vi "Get Minimum Import Pulse Width (clocks).vi"(0 "import signal":T1, 2 "acq":refnum<class "niUSRP DSP v2 FPGA.lvclass">=refnum) -> (4 "minimum import pulse width (clocks)":u16)   [LabVIEW 2023]
doc: "this setting determines how long the minimum pulse duration is for an exported signal. to calculate what the value is in seconds take the reciprocal of the ADC/DAC rate (seconds per clock tick) and multiply by number of clocks (min event pulse width)."
uses:
  <vilib>/rvi/DataTransferAndStorage/Container/XNode/niFpgaContainer.xnode
  <vilib>/rvi/DataTransferAndStorage/Register/Emulation/niFpgaRegisterEmulationRefIn.vi
  <instrlib>/niVST/Reference FPGA/FPGA/ACQ DSP/niUSRP DSP v2 FPGA.lvclass
  <instrlib>/niVST/Reference FPGA/FPGA/Acquisition/v1/Registers/Public/Typedefs/Imported Signals.ctl
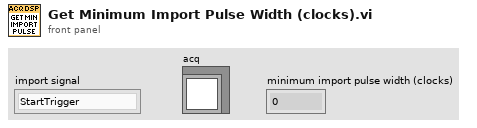
[diagram p1: front panel]
types:
  T1 = typedef "niVST Acquisition Registers v1 FPGA.lvclass/Imported Signals.ctl" = enum16{"StartTrigger", "RefTrigger", "AdvTrigger", "Configuration List Step Trigger", "Timer Start Trigger"}
  T2 = typedef "niUSRP DSP v2 FPGA.lvclass/DSP Shared Regs.ctl" = cluster{"rfsa.abort":refnum<k21>, "reset":refnum<k21>, "reset.done":refnum<k21>, "inject data into path":refnum<k21>, "data has entered path":refnum<k21>, "ADC overrange I":refnum<k21>, "ADC overrange Q":refnum<k21>, "ADC overrange.clear":refnum<k21>, "overflow":refnum<k21>, "overflow.clear":refnum<k21>, "pipeline delay":refnum<k21>, "group delay (output samples)":refnum<k21>, "dynamic delay.data clock ticks":refnum<k21>, "dynamic delay.samples":refnum<k21>, "scale data by 2":refnum<k21>, "bypass additional group delay":refnum<k21>, "debug.use wrapback data":refnum<k21>}
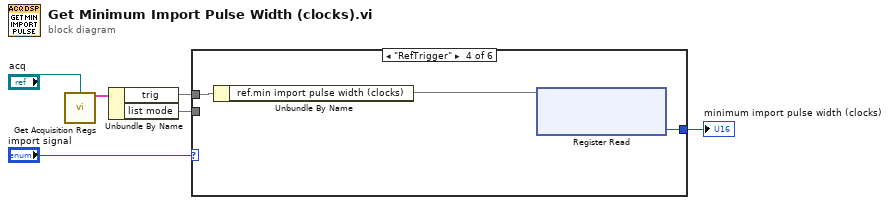
[diagram p0: block diagram]
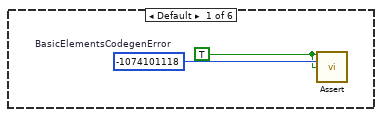
[diagram p2: hidden frame]
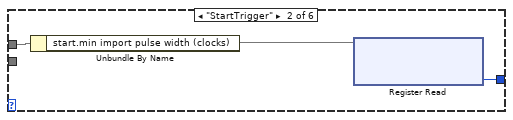
[diagram p3: hidden frame]
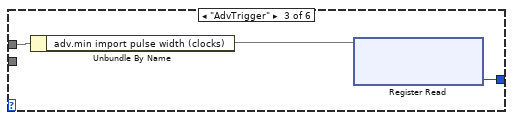
[diagram p4: hidden frame]
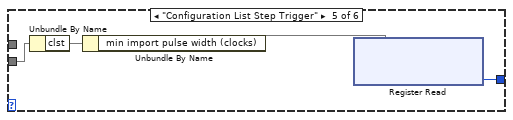
[diagram p5: hidden frame]
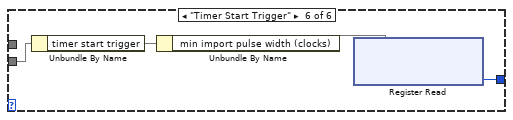
[diagram p6: hidden frame]
diagram:
  n1 = call-dynamic "Get Acquisition Regs.vi"("acq"="acq") -> ("dsp"=w3:T2)  [unwired: 14 in]
  n2 = Unbundle By Name(w3) -> ("trig"=w4, "list mode"=w1)
  n3 = case shown="\"RefTrigger\"" "import signal" {
    tunnel: [_ w10 w13 w16 w18 w22] -> w6
    tunnel: w4 -> [_ w9 w12 w15 _ _]
    tunnel: w1 -> [_ _ _ _ w21 w25]
    frame Default {
      w7 = TRUE ("assert")
      w8 = -1074101118  # BasicElementsCodegenError
      n4 = call <instrlib>:"Assert.vi"("assert"=w7, "error code"=w8, "enable show error"=w7) -> ()  [unwired: 13 in]
    }
    frame "StartTrigger" {
      n5 = Unbundle By Name(w9) -> ("start.min import pulse width (clocks)"=w11)
      n6 = xnode ("Register Read")("Register In"=w11) -> ("Data"=w10:u16)  [unwired: 1 out]
    }
    frame "AdvTrigger" {
      n7 = Unbundle By Name(w12) -> ("adv.min import pulse width (clocks)"=w14)
      n8 = xnode ("Register Read")("Register In"=w14) -> ("Data"=w13:u16)  [unwired: 1 out]
    }
    frame "RefTrigger" {
      n9 = Unbundle By Name(w15) -> ("ref.min import pulse width (clocks)"=w17)
      n10 = xnode ("Register Read")("Register In"=w17) -> ("Data"=w16:u16)  [unwired: 1 out]
    }
    frame "Configuration List Step Trigger" {
      n11 = Unbundle By Name(w21) -> ("clst"=w20)
      n12 = Unbundle By Name(w20) -> ("min import pulse width (clocks)"=w19)
      n13 = xnode ("Register Read")("Register In"=w19) -> ("Data"=w18:u16)  [unwired: 1 out]
    }
    frame "Timer Start Trigger" {
      n14 = Unbundle By Name(w25) -> ("timer start trigger"=w24)
      n15 = Unbundle By Name(w24) -> ("min import pulse width (clocks)"=w23)
      n16 = xnode ("Register Read")("Register In"=w23) -> ("Data"=w22:u16)  [unwired: 1 out]
    }
  }
  "minimum import pulse width (clocks)" <- w6
